vi "Car3UDPmsg_compose.vi"(0 "sender_IPv4":string, 1 "data (bytes string)":string, 5 "sender_port":u16=16100, 7 "receiver_IPv4":string, 9 "receiver_port":u16=16100, 11 "error in (no error)":errorcluster, 12 "msg_type":u8=1) -> (4 "message_bytes":string, 15 "error out":errorcluster)   [LabVIEW 2020]
panel:
  # "Composes a CARIBIC-3 (A350) UDP message.\n\nInputs:\n- sender address IPv4 and port (leave IP blank for auto-detect)\n- receiver address IPv4 and port\n- message type\n- message data\n\nOutput:\n- byte string\n\nLabVIEW version:\n- written with LV 2020 f1"
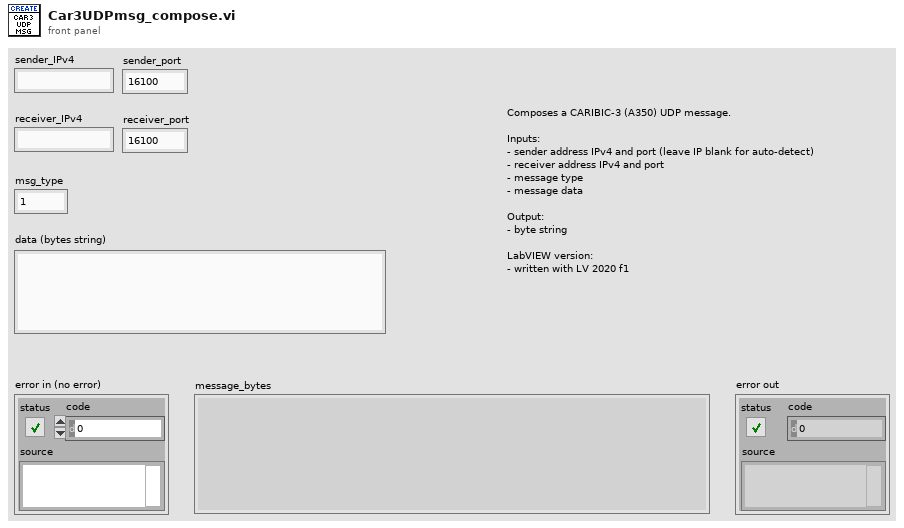
[diagram p1: front panel]
types:
  T1 = enum16{"big-endian, network order", "native, host order", "little-endian"}
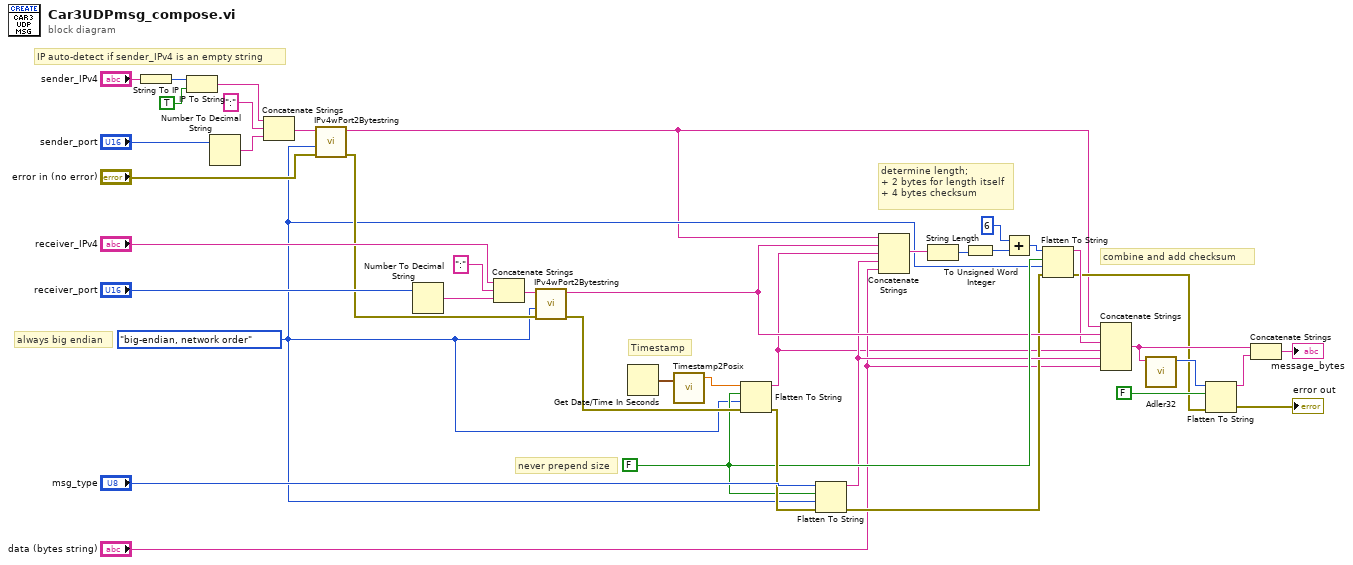
[diagram p0: block diagram]
diagram:
  w18 = T1."big-endian, network order" ("byte order (0:big-endian, network order)")
  w19 = FALSE ("prepend array or string size? (T)")
  # "combine and add checksum"
  # "determine length;\n+ 2 bytes for length itself\n+ 4 bytes checksum"
  # "never prepend size"
  # "always big endian"
  # "IP auto-detect if sender_IPv4 is an empty string"
  # "Timestamp"
  n1 = String To IP(1:"sender_IPv4") -> (0:w41:u32)
  n2 = IP To String(1:TRUE ("dot notation? (F)"), 2:w41) -> (0:w39:string)
  n3 = Number To Decimal String(number="sender_port") -> (decimal integer string=w37:string)  [unwired: 1 in]
  n4 = Concatenate Strings(w39, ":" ("string"), w37) -> (w34:string)
  n5 = call "IPv4wPort2Bytestring.vi"("error in"="error in (no error)", "byte order (0:big-endian, network order)"=w18, "ip address : port"=w34) -> ("error out"=w24:errorcluster, "byte string"=w5:string)  [unwired: 7 in]
  n6 = Number To Decimal String(number="receiver_port") -> (decimal integer string=w31:string)  [unwired: 1 in]
  n7 = Concatenate Strings("receiver_IPv4", ":" ("string"), w31) -> (w33:string)
  n8 = call "IPv4wPort2Bytestring.vi"("error in"=w24, "byte order (0:big-endian, network order)"=w18, "ip address : port"=w33) -> ("error out"=w23:errorcluster, "byte string"=w12:string)  [unwired: 7 in]
  n9 = Get Date/Time In Seconds() -> (seconds since 1Jan1904=w28:timestamp)
  n10 = call "Timestamp2Posix.vi"("timestamp"=w28) -> ("POSIX"=w27:dbl)  [unwired: 4 in]
  n11 = Flatten To String(anything=w27, prepend array or string size? (T)=w19, byte order (0:big-endian, network order)=w18, error in (no error)=w23) -> (data string=w4:string, error out=w22:errorcluster)  [unwired: 1 out]
  n12 = Flatten To String(anything="msg_type", prepend array or string size? (T)=w19, byte order (0:big-endian, network order)=w18, error in (no error)=w22) -> (data string=w10:string, error out=w7:errorcluster)  [unwired: 1 out]
  n13 = Concatenate Strings(w5, w12, w4, w10, "data (bytes string)") -> (w21:string)
  n14 = String Length(string=w21) -> (length=w20:i32)
  n15 = To Unsigned Word Integer(number=w20) -> (unsigned 16bit integer=w3:u16)
  n16 = Add(x=u16 6, y=w3) -> (x+y=w2:u16)
  n17 = Flatten To String(anything=w2, prepend array or string size? (T)=w19, byte order (0:big-endian, network order)=w18, error in (no error)=w7) -> (data string=w11:string, error out=w8:errorcluster)  [unwired: 1 out]
  n18 = Concatenate Strings(w5, w12, w11, w4, w10, "data (bytes string)") -> (w15:string)
  n19 = call "Adler32.vi"("input_string"=w15) -> ("Adler32"=w14:u32)  [unwired: 10 in]
  n20 = Flatten To String(anything=w14, prepend array or string size? (T)=FALSE, error in (no error)=w8) -> (data string=w16:string, error out=→"error out":errorcluster)  [unwired: 1 in, 1 out]
  n21 = Concatenate Strings(w15, w16) -> (→"message_bytes":string)
